vi "TableName2FolderPace.vi"(2 "TableName":string) -> (6 "FolderPace":T1)   [LabVIEW 2020, in "Sgraph_lib_V1.lvlib" / "DBAL-BIN.lvclass"]
uses:
  DBAL-BIN.lvclass
  BinFolderPace.ctl
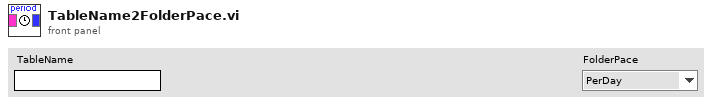
[diagram p1: front panel]
types:
  T1 = typedef "Sgraph_lib_V1.lvlib/DBAL-BIN.lvclass/BinFolderPace.ctl" = enum16{"PerDay", "PerWeek", "PerYear"}
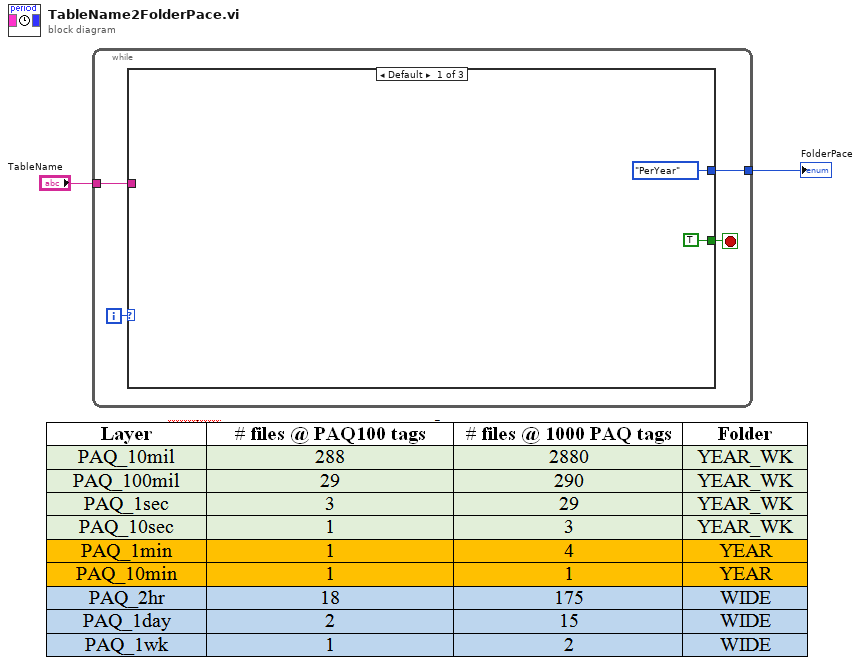
[diagram p0: block diagram]
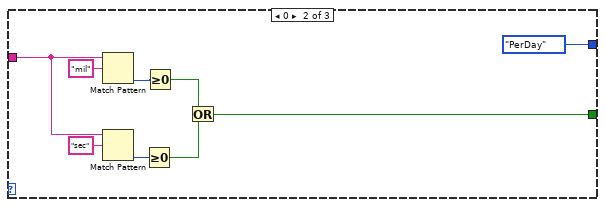
[diagram p2: hidden frame]
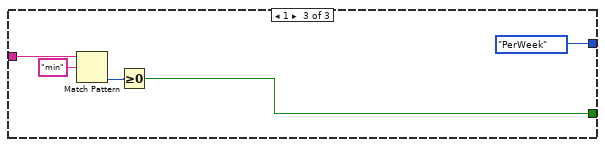
[diagram p3: hidden frame]
diagram:
  n1 = while {
    tunnel: "TableName" -> [w5]
    tunnel: [w3] -> w1
    i -> [w6]
    stop <- w4 stop-if-true
    n2 = case shown="Default" w6 {
      tunnel: w5 -> [_ w15 w20]
      tunnel: [TRUE w10 w19] -> w4
      tunnel: [BinFolderPace."PerYear" ("FolderPace") BinFolderPace."PerDay" ("FolderPace") BinFolderPace."PerWeek" ("FolderPace")] -> w3
      frame Default {
      }
      frame 0 {
        n3 = Match Pattern(string=w15, regular expression="mil") -> (offset past match=w14:i32)  [unwired: 1 in, 3 out]
        n4 = Match Pattern(string=w15, regular expression="sec") -> (offset past match=w13:i32)  [unwired: 1 in, 3 out]
        n5 = Greater Or Equal To 0?(x=w13) -> (x >= 0?=w11:bool)
        n6 = Greater Or Equal To 0?(x=w14) -> (x >= 0?=w12:bool)
        n7 = Or(x=w12, y=w11) -> (x .or. y?=w10:bool)
      }
      frame 1 {
        n8 = Match Pattern(string=w20, regular expression="min") -> (offset past match=w22:i32)  [unwired: 1 in, 3 out]
        n9 = Greater Or Equal To 0?(x=w22) -> (x >= 0?=w19:bool)
      }
    }
  }
  "FolderPace" <- w1
